vi "Actor Setup.vi"(10 "Actor":refnum<class "Actor.lvclass">, 11 "Dev Actor in":refnum<class "Dev Actor.lvclass">) -> (3 "Dev Actor out":refnum<class "Dev Actor.lvclass">)   [LabVIEW 2021, in "Dev Actor.lvlib" / "Dev Actor.lvclass"]
uses:
  Dev Actor.lvclass
  <vilib>/jettl/jettl/Actor/Actor/Actor.lvclass
  Dev Actor Panel/Dev Actor Panel.lvclass
  C:/git/Dev-Actor/src/Panel/Panel.lvclass
  Dev Actor.lvclass/Dev Actor.ctl
  Panel Create/Panel Create Msg Strategy/Panel Create Msg Strategy.lvclass
  C:/Program Files/National Instruments/LabVIEW 2021/vi.lib/jettl/jettl/Actor/Msg/Msg.lvclass
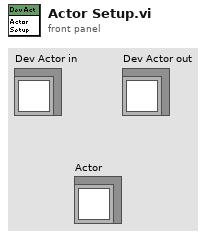
[diagram p1: front panel]
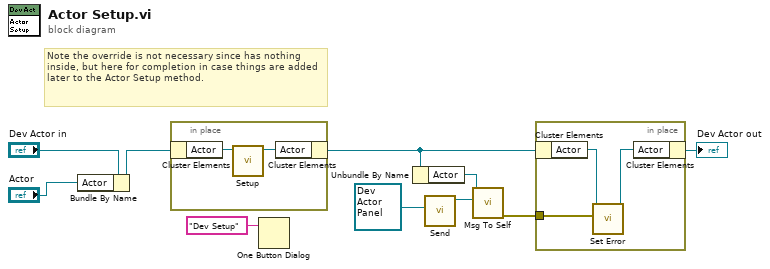
[diagram p0: block diagram]
diagram:
  # "Note the override is not necessary since has nothing inside, but here for completion in case things are added later to the Actor Setup method."
  n1 = Bundle By Name(cluster="Dev Actor in", "Actor"="Actor") -> (w8:refnum<class "Dev Actor.lvclass">)
  n2 = in-place {
    n3 = in-place-cluster #1(w8) -> ("Actor"=w11:refnum<class "Actor.lvclass">)
    n4 = call-dynamic "Setup.vi"("Actor in"=w11) -> ("Actor out"=w12:refnum<class "Actor.lvclass">)  [unwired: 10 in]
    n5 = in-place-cluster #1("Actor"=w12) -> (w6:refnum<class "Dev Actor.lvclass">)
  }
  n6 = One Button Dialog(message="Dev Setup") -> ()  [unwired: 1 in, 1 out]
  n7 = Unbundle By Name(w6) -> ("Actor"=w5:refnum<class "Actor.lvclass">)
  n8 = call "Send.vi"("Panel"=refnum<class "Dev Actor Panel.lvclass"> refnum ("Dev Actor Panel.lvclass")) -> ("Panel Create Msg Strategy out"=w3:refnum<class "Panel Create Msg Strategy.lvclass">)  [unwired: 10 in]
  n9 = call-dynamic "Msg To Self.vi"("Msg"=w3, "Actor in"=w5) -> ("error out"=w4:errorcluster)  [unwired: 9 in]
  n10 = in-place {
    in-place-border: w4 -> [w13]
    n11 = in-place-cluster #2(w6) -> ("Actor"=w15:refnum<class "Actor.lvclass">)
    n12 = call-dynamic "Set Error.vi"("Error"=w13, "Set Error in"=w15) -> ("Set Error out"=w14:refnum<class "Actor.lvclass">)  [unwired: 9 in]
    n13 = in-place-cluster #2("Actor"=w14) -> (→"Dev Actor out":refnum<class "Dev Actor.lvclass">)
  }
